vi "get buckets for graph averaging.vi"(1 "interval":dbl, 2 "Numeric":dbl, 3 "Numeric 2":dbl) -> (0 "Array":dbl[](array[numeric]))   [LabVIEW 2009]
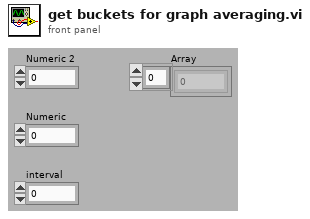
[diagram p1: front panel]
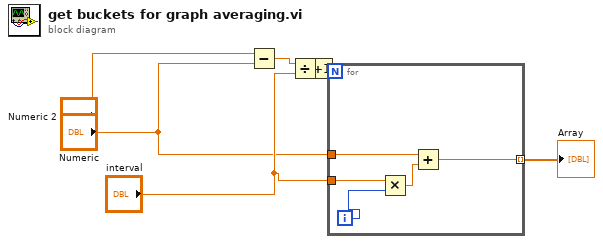
[diagram p0: block diagram]
diagram:
  n1 = Subtract(x="Numeric 2", y="Numeric") -> (x-y=w3:dbl)
  n2 = Divide(x=w3, y="interval") -> (x/y=w5:dbl)
  n3 = Increment(x=w5) -> (x+1=w7:dbl)
  n4 = for {
    N: w7 -> [_]
    tunnel: "interval" -> [w12]
    tunnel: "Numeric" -> [w9]
    tunnel: [w8] -> w6 mode=indexing
    i -> [w11]
    n5 = Multiply(x=w12, y=w11) -> (x*y=w10:dbl)
    n6 = Add(x=w9, y=w10) -> (x+y=w8:dbl)
  }
  "Array" <- w6
